vi "test Loopback RT to RT with Start Stop and Status.vi"(8 "error in":errorcluster, 11 "TestCase in":refnum<class "Loopback.lvclass">) -> (0 "error out":errorcluster, 3 "TestCase out":refnum<class "Loopback.lvclass">)   [LabVIEW 2020, in "Loopback.lvclass"]
uses:
  Loopback.lvclass
  C:/Git/niveristand-custom-device-testing-tools/VeriStandTestCase/VeriStandTestCase.lvclass
  <vilib>/numeric/Random Number (Range) U64.vi
  1571aa8d-489e-4c94-925a-256c0ab49a50.vi
  <vilib>/numeric/sub_Random U32.vi
  <vilib>/NI VeriStand/Execution/Workspace/NI VeriStand - Get Multiple Channel Values.vi
  <vilib>/NI VeriStand/Execution/Workspace/NI VeriStand - Set Single Channel Value.vi
  <vilib>/NI VeriStand/Execution/Workspace/NI VeriStand - Set Multiple Channel Values.vi
  <vilib>/addons/_JKI Toolkits/VI Tester/TestCase.llb/TestCase.lvclass
  <vilib>/NI VeriStand/Execution/Workspace/NI_VS Workspace ExecutionAPI.lvlib
  niveristand-custom-device-testing-tools/VeriStandTestUtilities/VeriStandTestUtilities.lvlib
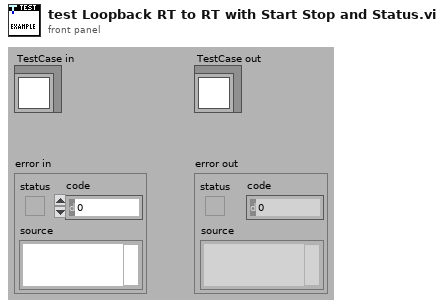
[diagram p1: front panel]
types:
  T1 = typedef "NI_VS Workspace ExecutionAPI.lvlib/WorkspaceAPI.ctl" = refnum<k24>
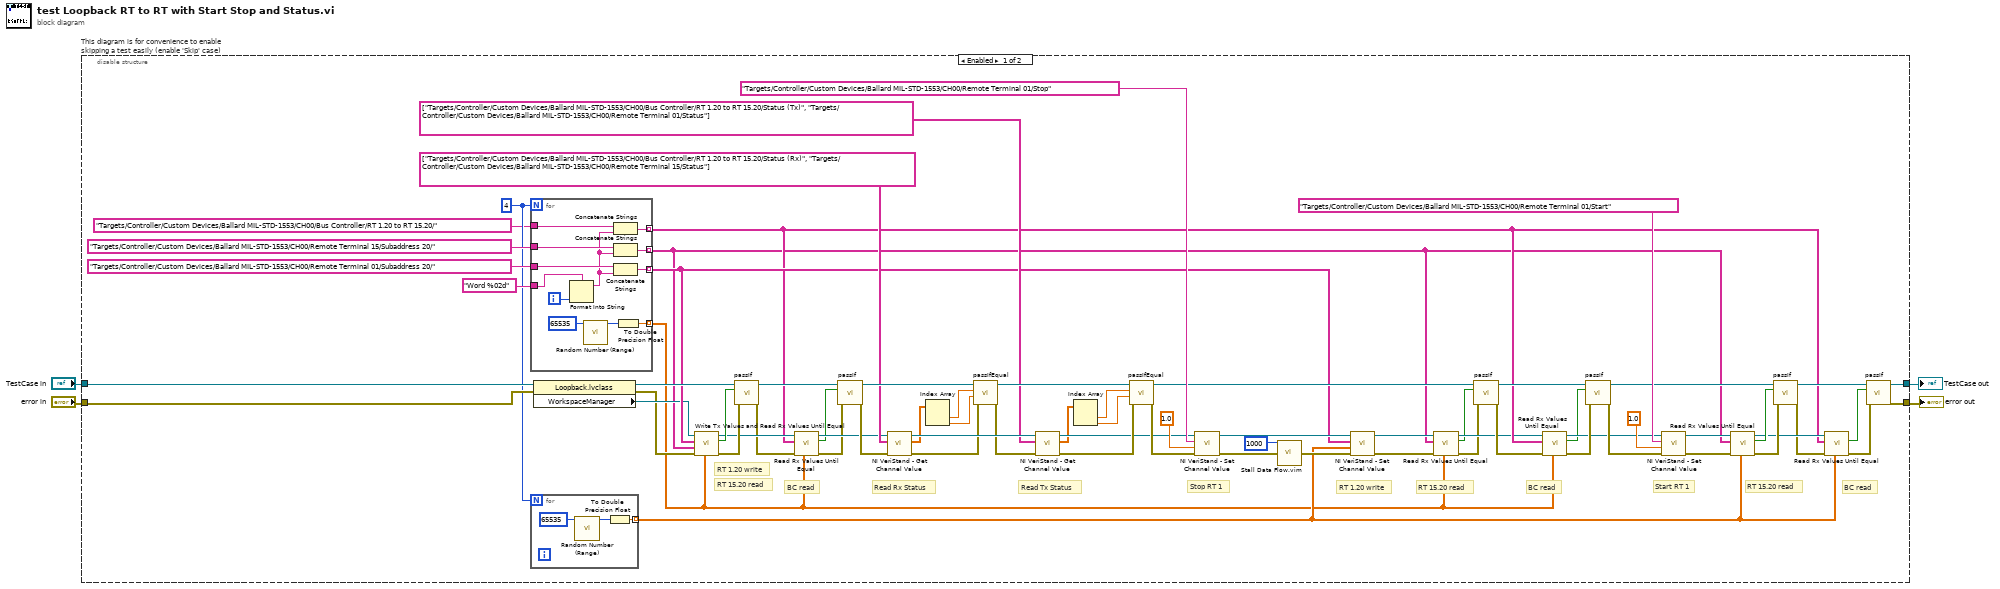
[diagram p0: block diagram]
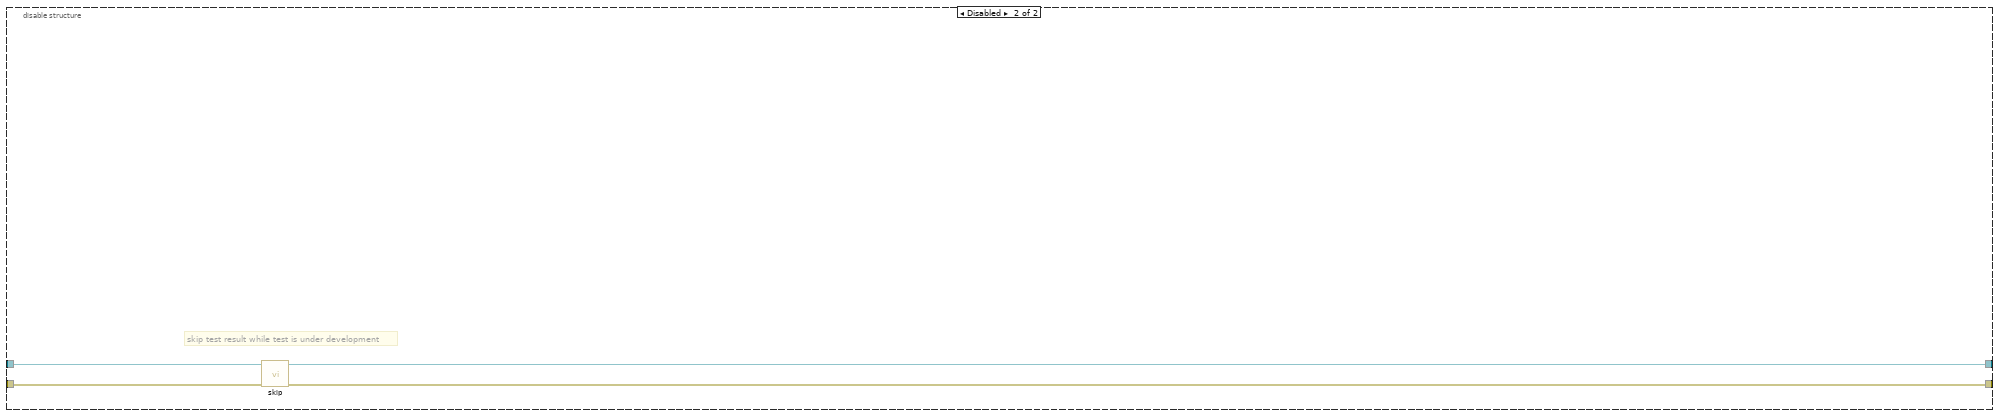
[diagram p2: hidden frame]
diagram:
  n1 = disable-structure "This diagram is for convenience to enable skipping a test easily (enable 'Skip' case)" shown="Enabled" {
    disable-tunnel: "TestCase in" -> [w75 w95]
    disable-tunnel: [w57 w93] -> w1
    disable-tunnel: [w58 w94] -> w3
    disable-tunnel: "error in" -> [w72 w92]
    frame Enabled {
      w62 = 4
      # "Read Tx Status"
      # "Read Rx Status"
      # "BC read"
      # "RT 15.20 read"
      # "BC read"
      # "RT 15.20 read"
      # "RT 1.20 write"
      # "BC read"
      # "RT 15.20 read"
      # "RT 1.20 write"
      # "Start RT 1"
      # "Stop RT 1"
      n2 = for {
        N: w62 -> [_]
        tunnel: "Targets/Controller/Custom Devices/Ballard MIL-STD-1553/CH00/Remote Terminal 01/Subaddress 20/" ("Channel") -> [w87]
        tunnel: [w88] -> w35 mode=indexing
        tunnel: "Targets/Controller/Custom Devices/Ballard MIL-STD-1553/CH00/Remote Terminal 15/Subaddress 20/" ("Channel") -> [w86]
        tunnel: [w85] -> w9 mode=indexing
        tunnel: "Word %02d" -> [w77]
        tunnel: [w81] -> w8 mode=indexing
        tunnel: "Targets/Controller/Custom Devices/Ballard MIL-STD-1553/CH00/Bus Controller/RT 1.20 to RT 15.20/" ("Channel") -> [w80]
        tunnel: [w78] -> w16 mode=indexing
        i -> [w84]
        n3 = Format Into String(format string=w77, w84) -> (resulting string=w79:string)  [unwired: 2 in, 1 out]
        n4 = call-poly <vilib>:"Random Number (Range).vi"("upper bound (100)"=u64 65535) -> ("number"=w83:u64)  [unwired: 10 in]
        n5 = Concatenate Strings(w80, w79) -> (w78:string)
        n6 = Concatenate Strings(w86, w79) -> (w85:string)
        n7 = Concatenate Strings(w87, w79) -> (w88:string)
        n8 = To Double Precision Float(number=w83) -> (double precision float=w81:dbl)
      }
      n9 = for {
        N: w62 -> [_]
        tunnel: [w89] -> w18 mode=indexing
        n10 = call-poly <vilib>:"Random Number (Range).vi"("upper bound (100)"=u64 65535) -> ("number"=w90:u64)  [unwired: 10 in]
        n11 = To Double Precision Float(number=w90) -> (double precision float=w89:dbl)
      }
      n12 = property class="Loopback.lvclass"(reference=w75, error in=w72) -> (reference out=w76:refnum<class "Loopback.lvclass">, error out=w33:errorcluster, "WorkspaceManager"=w34:T1)
      n13 = call "Write Tx Values and Read Rx Values Until Equal.vi"("Tx values"=w8, "error in"=w33, "Rx aliases"=w9, "Tx aliases"=w35, "workspace manager in"=w34) -> ("error out"=w32:errorcluster, "values equal"=w31:bool, "workspace manager out"=w30:T1)  [unwired: 4 in]
      n14 = call-dynamic "passIf.vi"("error in (no error)"=w32, "pass"=w31, "TestCase in"=w76) -> ("error out"=w29:errorcluster, "TestCase out"=w60:refnum<class "Loopback.lvclass">)  [unwired: 7 in]
      n15 = call "Read Rx Values Until Equal.vi"("expected values"=w8, "error in"=w29, "Rx aliases"=w16, "workspace manager in"=w30) -> ("error out"=w27:errorcluster, "values equal expected"=w26:bool, "workspace manager out"=w28:T1)  [unwired: 5 in]
      n16 = call-dynamic "passIf.vi"("error in (no error)"=w27, "pass"=w26, "TestCase in"=w60) -> ("error out"=w48:errorcluster, "TestCase out"=w47:refnum<class "Loopback.lvclass">)  [unwired: 7 in]
      n17 = call-poly <vilib>:"NI VeriStand - Get Channel Value.vi"("error in (no error)"=w48, "Channels"=string[] ["Targets/Controller/Custom Devices/Ballard MIL-STD-1553/CH00/Bus Controller/RT 1.20 to RT 15.20/Status (Rx)", "Targets/Controller/Custom Devices/Ballard MIL-STD-1553/CH00/Remote Terminal 15/Status"], "WorkspaceManager in"=w28) -> ("error out"=w49:errorcluster, "Values"=w40:dbl[], "WorkspaceManager out"=w53:T1)  [unwired: 6 in]
      n18 = Index Array(array=w40) -> (element #1=w39:dbl, element #2=w38:dbl)  [unwired: 2 in]
      n19 = call-dynamic "passIfEqual.vi"("error in (no error)"=w49, "y"=w38, "x"=w39, "TestCase in"=w47) -> ("error out"=w51:errorcluster, "TestCase out"=w52:refnum<class "Loopback.lvclass">)  [unwired: 6 in]
      n20 = call-poly <vilib>:"NI VeriStand - Get Channel Value.vi"("error in (no error)"=w51, "Channels"=string[] ["Targets/Controller/Custom Devices/Ballard MIL-STD-1553/CH00/Bus Controller/RT 1.20 to RT 15.20/Status (Tx)", "Targets/Controller/Custom Devices/Ballard MIL-STD-1553/CH00/Remote Terminal 01/Status"], "WorkspaceManager in"=w53) -> ("error out"=w50:errorcluster, "Values"=w43:dbl[], "WorkspaceManager out"=w45:T1)  [unwired: 6 in]
      n21 = Index Array(array=w43) -> (element #1=w42:dbl, element #2=w41:dbl)  [unwired: 2 in]
      n22 = call-dynamic "passIfEqual.vi"("error in (no error)"=w50, "y"=w41, "x"=w42, "TestCase in"=w52) -> ("error out"=w46:errorcluster, "TestCase out"=w44:refnum<class "Loopback.lvclass">)  [unwired: 6 in]
      n23 = call-poly <vilib>:"NI VeriStand - Set Channel Value.vi"("error in (no error)"=w46, "Value"=1.0, "Channel"="Targets/Controller/Custom Devices/Ballard MIL-STD-1553/CH00/Remote Terminal 01/Stop", "WorkspaceManager in"=w45) -> ("error out"=w64:errorcluster, "WorkspaceManager out"=w68:T1)  [unwired: 6 in]
      n24 = call "Stall Data Flow.vim"("value in"=w64, "milliseconds to wait"=u32 1000) -> ("value out"=w63:errorcluster)  [unwired: 1 out]
      n25 = call-poly <vilib>:"NI VeriStand - Set Channel Value.vi"("error in (no error)"=w63, "Values"=w18, "Channels"=w35, "WorkspaceManager in"=w68) -> ("error out"=w10:errorcluster, "WorkspaceManager out"=w11:T1)  [unwired: 6 in]
      n26 = call "Read Rx Values Until Equal.vi"("expected values"=w8, "error in"=w10, "Rx aliases"=w9, "workspace manager in"=w11) -> ("error out"=w6:errorcluster, "values equal expected"=w5:bool, "workspace manager out"=w7:T1)  [unwired: 5 in]
      n27 = call-dynamic "passIf.vi"("error in (no error)"=w6, "pass"=w5, "TestCase in"=w44) -> ("error out"=w15:errorcluster, "TestCase out"=w55:refnum<class "Loopback.lvclass">)  [unwired: 7 in]
      n28 = call "Read Rx Values Until Equal.vi"("expected values"=w8, "error in"=w15, "Rx aliases"=w16, "workspace manager in"=w7) -> ("error out"=w14:errorcluster, "values equal expected"=w12:bool, "workspace manager out"=w13:T1)  [unwired: 5 in]
      n29 = call-dynamic "passIf.vi"("error in (no error)"=w14, "pass"=w12, "TestCase in"=w55) -> ("error out"=w56:errorcluster, "TestCase out"=w54:refnum<class "Loopback.lvclass">)  [unwired: 7 in]
      n30 = call-poly <vilib>:"NI VeriStand - Set Channel Value.vi"("error in (no error)"=w56, "Value"=1.0, "Channel"="Targets/Controller/Custom Devices/Ballard MIL-STD-1553/CH00/Remote Terminal 01/Start", "WorkspaceManager in"=w13) -> ("error out"=w24:errorcluster, "WorkspaceManager out"=w25:T1)  [unwired: 6 in]
      n31 = call "Read Rx Values Until Equal.vi"("expected values"=w18, "error in"=w24, "Rx aliases"=w9, "workspace manager in"=w25) -> ("error out"=w22:errorcluster, "values equal expected"=w23:bool, "workspace manager out"=w21:T1)  [unwired: 5 in]
      n32 = call-dynamic "passIf.vi"("error in (no error)"=w22, "pass"=w23, "TestCase in"=w54) -> ("error out"=w20:errorcluster, "TestCase out"=w59:refnum<class "Loopback.lvclass">)  [unwired: 7 in]
      n33 = call "Read Rx Values Until Equal.vi"("expected values"=w18, "error in"=w20, "Rx aliases"=w16, "workspace manager in"=w21) -> ("error out"=w19:errorcluster, "values equal expected"=w17:bool)  [unwired: 5 in, 1 out]
      n34 = call-dynamic "passIf.vi"("error in (no error)"=w19, "pass"=w17, "TestCase in"=w59) -> ("error out"=w58:errorcluster, "TestCase out"=w57:refnum<class "Loopback.lvclass">)  [unwired: 7 in]
    }
    frame Disabled {
      # "skip test result while test is under development"
      n35 = call <vilib>:"skip.vi"("error in (no error)"=w92, "TestCase in"=w95) -> ("error out"=w94:errorcluster, "TestCase out"=w93:refnum<class "Loopback.lvclass">)  [unwired: 8 in]
    }
  }
  "error out" <- w3
  "TestCase out" <- w1
